vi "Create.vi"(5 "Property in":refnum<class "Property.lvclass">, 8 "error in (no error)":errorcluster, 9 "Value":string, 10 "Name":string) -> (0 "error out":errorcluster, 3 "Property":refnum<class "Property.lvclass">)   [LabVIEW 2013, in "JUnit XML.lvlib" / "Property.lvclass"]
uses:
  Property.lvclass
  Property.lvclass/Property.ctl
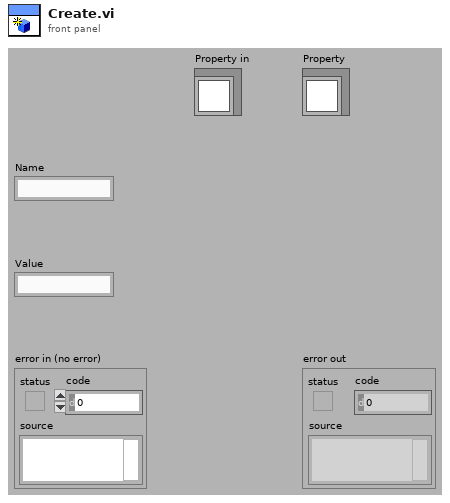
[diagram p1: front panel]
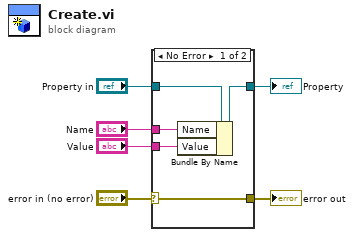
[diagram p0: block diagram]
diagram:
  n1 = case shown="No Error" "error in (no error)" {
    selector: "error in (no error)" -> [w11 w13]
    tunnel: [w11 w13] -> w5
    tunnel: [w9 w12] -> w3
    tunnel: "Property in" -> [w10 w12]
    tunnel: "Name" -> [w8 _]
    tunnel: "Value" -> [w7 _]
    frame No Error {
      n2 = Bundle By Name(cluster=w10, "Name"=w8, "Value"=w7) -> (w9:refnum<class "Property.lvclass">)
    }
    frame Error {
    }
  }
  "error out" <- w5
  "Property" <- w3
